vi "Py - Cs Total.vi"(8 "error in":errorcluster, 10 "En":dbl, 11 "Z":i32) -> (0 "error out":errorcluster, 3 "Cs Total":dbl)   [LabVIEW 2023]
uses:
  global python version.vi
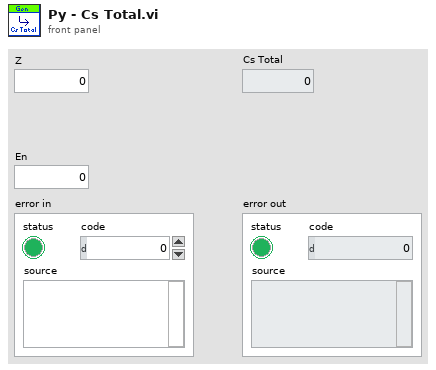
[diagram p1: front panel]
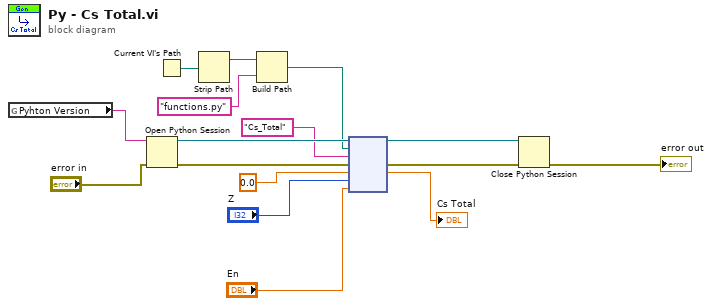
[diagram p0: block diagram]
diagram:
  n1 = global read "global python version.vi" "Pyhton Version"() -> (w4:string)
  n2 = Open Python Session(python version=w4, 3:"error in") -> (session out=w13:refnum<k35>, error out=w10:errorcluster)  [unwired: 1 in]
  n3 = Current VI's Path() -> (path=w15:path)
  n4 = Strip Path(path=w15) -> (stripped path=w14:path)  [unwired: 1 out]
  n5 = Build Path(base path=w14, name or relative path="functions.py") -> (appended path=w6:path)
  n6 = node(w13, w6, "Cs_Total", w10, 0.0, "Z", "En") -> (w12:refnum<k35>, w11:errorcluster, →"Cs Total":dbl)  [unwired: 2 in, 2 out]
  n7 = Close Python Session(session in=w12, error in=w11) -> (11:→"error out":errorcluster)
